vi "DosagesQueueHandler.vi"(8 "error in (no error)":errorcluster, 10 "DosagesQueueName":string, 11 "CurrentTime":timestamp) -> (0 "error out":errorcluster, 2 "AppliedDosage":T1, 3 "Sucess":bool)   [LabVIEW 2019]
uses:
  DrugDosageTimeStampReference.ctl
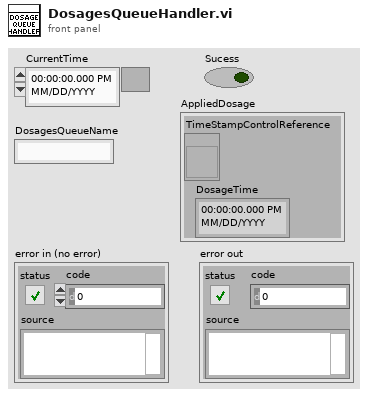
[diagram p1: front panel]
types:
  T1 = typedef "DrugDosageTimeStampReference.ctl" = cluster{"TimeStampControlReference":refnum<vi>, "DosageTime":timestamp}
  T2 = enum8{"Enabled", "Disabled", "Disabled and Grayed Out"}
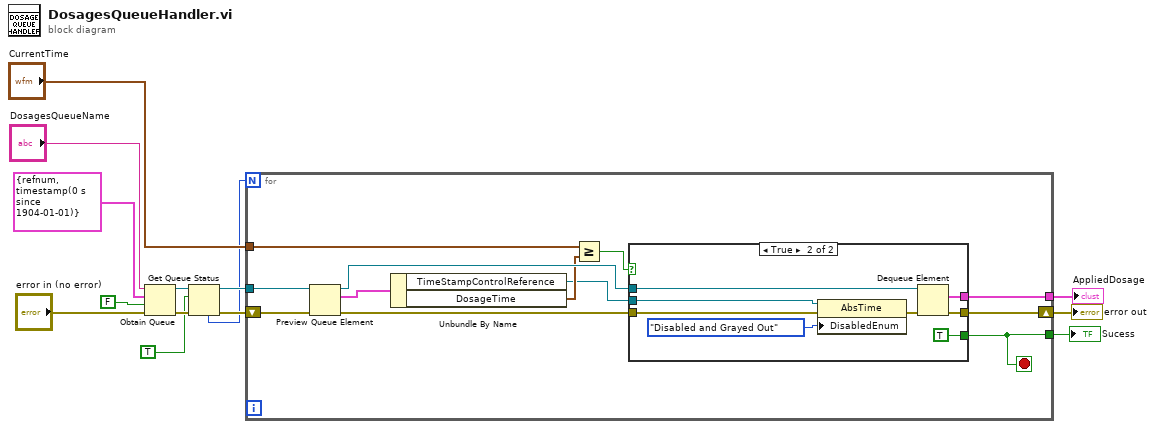
[diagram p0: block diagram]
diagram:
  n1 = Obtain Queue(name (unnamed)="DosagesQueueName", element data type=T1 {"TimeStampControlReference"=refnum, "DosageTime"=timestamp(0 s since 1904-01-01)}, create if not found? (T)=FALSE, error in (no error)="error in (no error)") -> (queue out=w6:refnum<queue>, error out=w5:errorcluster)  [unwired: 1 in, 1 out]
  n2 = Get Queue Status(queue=w6, return elements? (F)=TRUE, error in (no error)=w5) -> (queue out=w3:refnum<queue>, error out=w4:errorcluster, # elements in queue=w1:i32)  [unwired: 5 out]
  n3 = for {
    N: w1 -> [_]
    tunnel: w3 -> [w25]
    tunnel: "CurrentTime" -> [w23]
    shift-right: [w20] -> w13
    shift-left: w4 -> [w26]
    tunnel: [w18] -> w12
    tunnel: [w19] -> w10
    stop <- w18 stop-if-true
    n4 = Preview Queue Element(queue=w25, error in (no error)=w26) -> (queue out=w22:refnum<queue>, element=w24:T1, error out=w21:errorcluster)  [unwired: 1 in, 1 out]
    n5 = Unbundle By Name(w24) -> ("TimeStampControlReference"=w16:refnum<vi>, "DosageTime"=w17:timestamp)
    n6 = Greater Or Equal?(x=w23, y=w17) -> (x >= y?=w15:bool)
    n7 = case shown="True" w15 {
      tunnel: w16 -> [_ w35]
      tunnel: w22 -> [_ w33]
      tunnel: w21 -> [w27 w32]
      tunnel: [w27 w30] -> w20
      tunnel: [_ w29] -> w19
      tunnel: [_ TRUE] -> w18
      frame False {
      }
      frame True {
        n8 = property class="AbsTime"(reference=w35, error in=w32, "DisabledEnum"=T2."Disabled and Grayed Out" ("Disabled")) -> (error out=w31:errorcluster)  [unwired: 1 out]
        n9 = Dequeue Element(queue=w33, error in (no error)=w31) -> (element=w29:T1, error out=w30:errorcluster)  [unwired: 1 in, 2 out]
      }
    }
  }
  "error out" <- w13
  "Sucess" <- w12
  "AppliedDosage" <- w10
